vi "Get Sensitivity Values.vi"(8 "error in (no error)":errorcluster, 11 "APU Setup File":T1) -> (0 "Error Out":errorcluster, 1 "Fan":dbl[](array[numeric]), 2 "GS":dbl[](array[numeric]), 3 "PS":dbl[](array[numeric]))   [LabVIEW 2018, in "Testing UI 3.lvlib"]
uses:
  Testing UI 3.lvlib
  Top Level/Shared Controls/APU Setup File.ctl
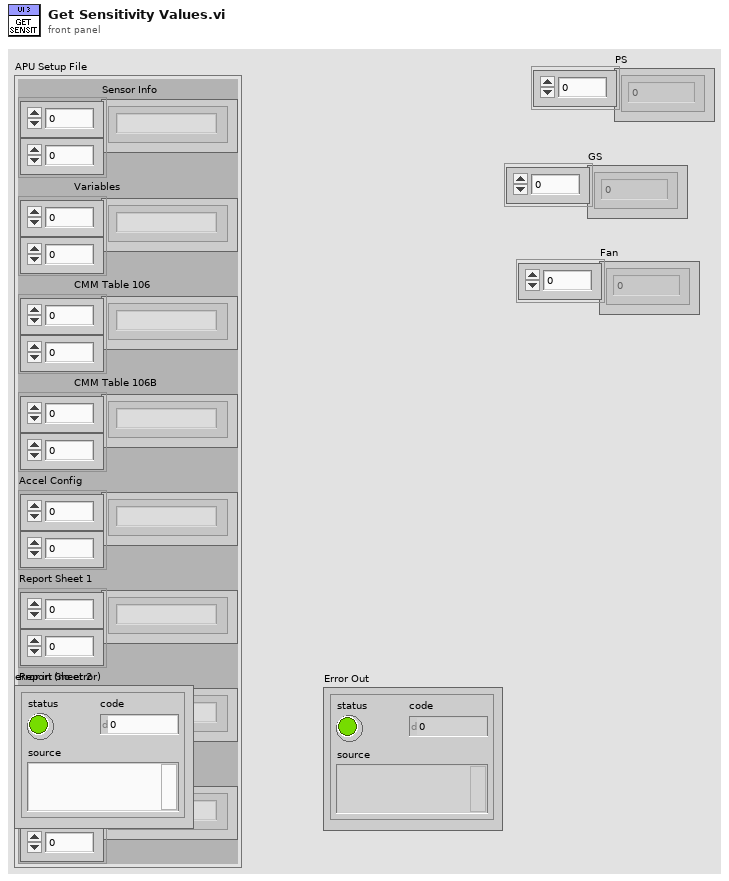
[diagram p1: front panel]
types:
  T1 = typedef "APU Setup File.ctl" = cluster{"Sensor Info":string[][], "Variables":string[][], "CMM Table 106":string[][], "CMM Table 106B ":string[][], "Accel Config":string[][], "Report Sheet 1":string[][], "Report Sheet 2":string[][], "Report Sheet 3":string[][]}
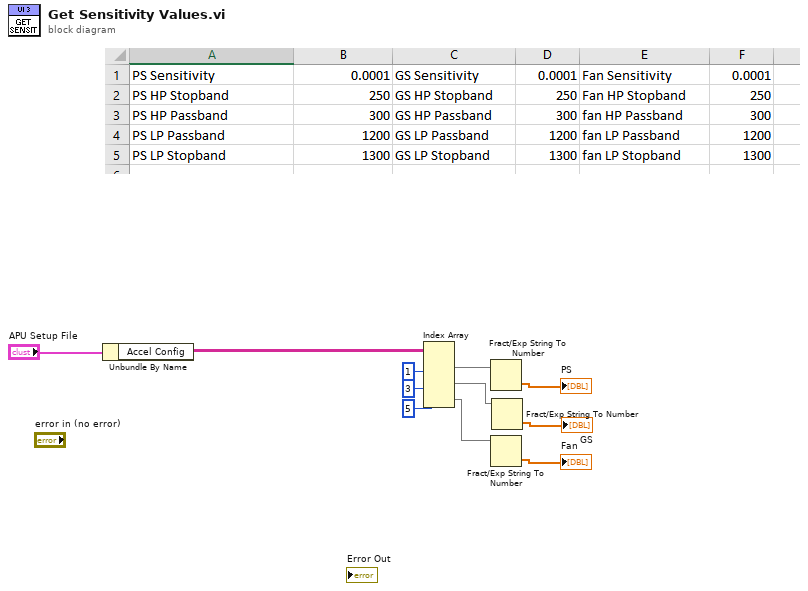
[diagram p0: block diagram]
diagram:
  n1 = Unbundle By Name("APU Setup File") -> ("Accel Config"=w9:string[][])
  n2 = Index Array(array=w9, index (col) #1=1 ("disabled index (col)"), index (col) #2=3 ("index (col)"), index (col) #3=5 ("index (col)")) -> (element #1=w8:string[], element #2=w4:string[], element #3=w1:string[])  [unwired: 3 in]
  n3 = Fract/Exp String To Number(string=w8) -> (number=→"PS":dbl[])  [unwired: 3 in, 1 out]
  n4 = Fract/Exp String To Number(string=w1) -> (number=→"Fan":dbl[])  [unwired: 3 in, 1 out]
  n5 = Fract/Exp String To Number(string=w4) -> (number=→"GS":dbl[])  [unwired: 3 in, 1 out]
